vi "Test DUT Trigger Self Test Broadcast.vi"(8 "error in (no error)":errorcluster, 11 "Device Under Test Test In":refnum<class "Device Under Test Test.lvclass">) -> (0 "error out":errorcluster, 3 "Device Under Test Test Out":refnum<class "Device Under Test Test.lvclass">)   [LabVIEW 2020, in "Device Under Test Test.lvclass"]
uses:
  Device Under Test Test.lvclass
  C:/Program Files (x86)/National Instruments/LabVIEW 2020/vi.lib/Astemes/LUnit/Test Case.lvclass
  Device Under Test/Device Under Test.lvclass
  C:/Program Files (x86)/National Instruments/LabVIEW 2020/vi.lib/Astemes/Triarc Framework/Process/Process.lvclass
  <vilib>/Astemes/Triarc Framework/Process/Process.lvclass/Process.ctl
  <vilib>/Astemes/LUnit/Test Case.lvclass/Test Case.ctl
  <vilib>/Astemes/Triarc Framework/Broadcast Event Helpers/Execution timer.vi
  <vilib>/Astemes/Triarc Framework/Process/Private/SubVIs/Wait for finish.vi
  <vilib>/Astemes/Triarc Framework/Process/Private/SubVIs/Set Lifecycle State.vi
  <vilib>/Astemes/Triarc Framework/Process/Protected/Messaging/Send Message.vi
  <vilib>/Astemes/LUnit/Core/LUnit Test Case/Private/Append Pass Result.vi
  <vilib>/Astemes/LUnit/Core/LUnit Test Case/Private/Append Fail Result.vi
  <vilib>/Astemes/Triarc Framework/Process/Private/SubVIs/Handle Debug Data.vi
  <vilib>/Astemes/LUnit/Core/LUnit Test Case/Private/Run In UI.vi
  <vilib>/Utility/error.llb/Clear Errors.vi
  <vilib>/Astemes/Triarc Framework/Support/Dequeue Broadcast Message.vi
  <vilib>/Astemes/Triarc Framework/Process/Public/Lifecycle/Get Lifecycle State.vi
  <vilib>/Utility/error.llb/Error Cluster From Error Code.vi
  <vilib>/Astemes/Triarc Framework/Callback/Callback.lvclass
  <vilib>/Astemes/Triarc Framework/Process/Process.lvclass
  <vilib>/Astemes/LUnit/Test Case.lvclass
  <vilib>/Astemes/Triarc Framework/Broadcast Event Helpers/Broadcast Event Helpers.lvlib
panel:
  out "Message Data":variant
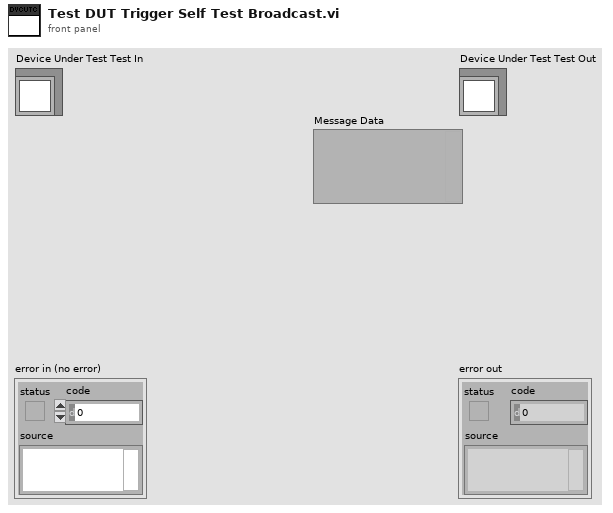
[diagram p1: front panel]
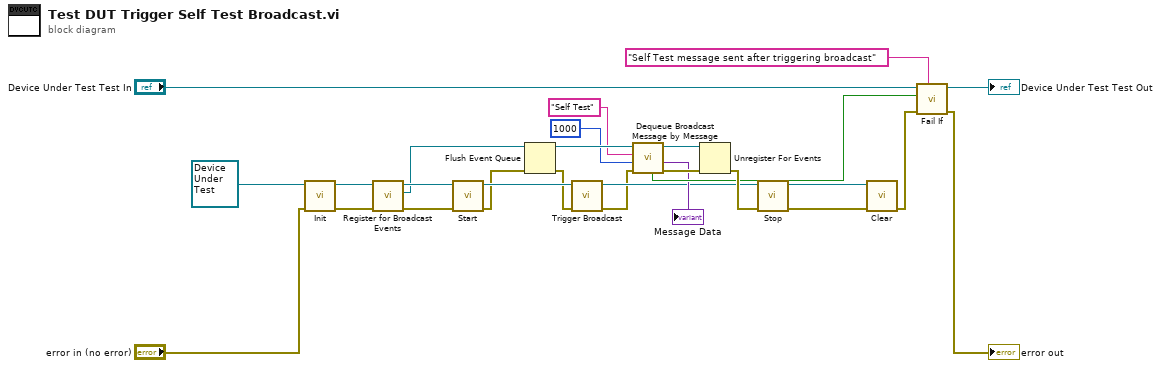
[diagram p0: block diagram]
diagram:
  n1 = call-dynamic "Init.vi"("error in (no error)"="error in (no error)", "View In"=refnum<class "Device Under Test.lvclass"> refnum ("Device Under Test.lvclass")) -> ("error out"=w22:errorcluster, "View Out"=w24:refnum<class "Device Under Test.lvclass">)  [unwired: 8 in]
  n2 = call <vilib>:"Register for Broadcast Events.vi"("error in (no error)"=w22, "Process In"=w24) -> ("error out"=w21:errorcluster, "Event Registration Refnum Out"=w13:refnum<event-registration>, "Process Out"=w23:refnum<class "Device Under Test.lvclass">)  [unwired: 7 in]
  n3 = call <vilib>:"Start.vi"("error in (no error)"=w21, "Process In"=w23) -> ("error out"=w3:errorcluster, "Process Out"=w5:refnum<class "Device Under Test.lvclass">)  [unwired: 7 in, 1 out]
  n4 = Flush Event Queue(0:w13, 3:w3) -> (8:w12:refnum<event-registration>, 11:w2:errorcluster)  [unwired: 4 in, 1 out]
  n5 = call <vilib>:"Trigger Broadcast.vi"("error in (no error)"=w2, "Process in"=w5) -> ("error out"=w1:errorcluster, "Process out"=w4:refnum<class "Device Under Test.lvclass">)  [unwired: 8 in]
  n6 = call <vilib>:"Dequeue Broadcast Message by Message.vi"("error in (no error)"=w1, "Timeout (-1)"=1000, "Message"="Self Test", "Event Registration Refnum"=w12) -> ("error out"=w14:errorcluster, "Message Data"=→"Message Data":variant, "Event Registration Refnum Out"=w10:refnum<event-registration>, "Timed Out?"=w8:bool)  [unwired: 3 in, 1 out]
  n7 = Unregister For Events(event registration refnum=w10, error in=w14) -> (error out=w11:errorcluster)
  n8 = call <vilib>:"Stop.vi"("error in (no error)"=w11, "Process In"=w4) -> ("error out"=w25:errorcluster, "Process Out"=w26:refnum<class "Device Under Test.lvclass">)  [unwired: 7 in, 1 out]
  n9 = call-dynamic "Clear.vi"("error in (no error)"=w25, "View In"=w26) -> ("error out"=w19:errorcluster)  [unwired: 9 in]
  n10 = call <vilib>:"Fail If.vi"("Description"="Self Test message sent after triggering broadcast", "error in (no error)"=w19, "Fail?"=w8, "LUnit Test Case In"="Device Under Test Test In") -> ("error out"=→"error out":errorcluster, "LUnit Test Case Out"=→"Device Under Test Test Out":refnum<class "Device Under Test Test.lvclass">)  [unwired: 6 in]
